vi "TOOLweb TRIGGER.vi"(4 "error in (no error)":errorcluster caption="Fehler (Eingang, kein Fehler)", 5 "IP-Adresse (localhost)":string="127.0.0.1", 7 "action":T2) -> (2 "trigger-Diagnose":T1, 3 "Trigger ausgeführt":bool)   [LabVIEW 2020, in "FT-IR.lvlib" / "TOOLweb Interface.lvlib"]
doc: "Ändert den Betriebszustand des Messgerätes durch Triggern einer Aktion \"action\" (start run, run once, stop run, pause run, resume run, take back). Der Trigger wird durch einen PollRequest an EVID 31..36 (je nach Aktion) ausgelöst. Nachher wird durch Polling der Variablen EVID30 (trigger-lastdatetime) verifiziert, ob der Trigger erfolgreich ausgeführt wurde.\n\n\"Trigger ausgeführt\" ist TRUE, wenn\n1) die Datum/Zeit in der Antwort einen Zeitpunkt nach dem Senden des PollRequests ergeben UND\n2) der Name der Aktion im Poll-Response mit der angeforderten Aktion übereinstimmt.\n\nDer Ausgangs-Cluster \"trigger-Diagnose\" ermöglicht eine weitere Fehlererkennung:\naction-name: die angeforderte Aktion\nlastname: die zuletzt erfolgreich ausgeführte Trigger-Aktion\nlastdatetime: der Zeitpunkt der zuletzt erfolgreich ausgeführten Aktion\nSystemzeit: der Zeitpunkt des Sendens der Trigger-Anforderung (PollRequest)"
uses:
  TOOLweb Interface.lvlib
  Trigger Aktionen.ctl
  Stoerungen/Stoerungen Messgeraet/Aktionen Kommunikation Stoerung.ctl
  TOOLweb Interface Hilfs-VIs.lvlib
  Stoerungen/Stoerungen.lvlib
  Typdefinitionen.lvlib
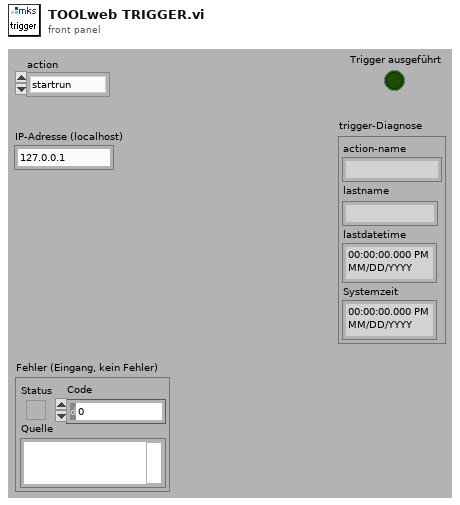
[diagram p1: front panel]
types:
  T1 = cluster{"action-name":string, "lastname":string, "lastdatetime":timestamp, "Systemzeit":timestamp}
  T2 = typedef "FT-IR.lvlib/TOOLweb Interface.lvlib/Typdefinitionen.lvlib/Trigger Aktionen.ctl" = enum16{"startrun", "runonce", "stoprun", "pauserun", "resumerun", "takeback"}
  T3 = typedef "Stoerungen.lvlib/Aktionen Kommunikation Stoerung.ctl" = enum16{"lesen", "init", "FT-IR Komm", "FT-IR Betriebsart", "FT-IR Hintergrund", "cRIO Komm", "PNS Komm", "Dichtheitstest", "Life Bit", "FTIR Komm AK", "PMA Komm", "FID Komm", "PMA Cal", "FID Ch4 Cal", "FID THC Cal", "Cal Timeout", "VFS 1 Komm", "VFS 2 Komm", "VFS 3 Komm", "VFS 4 Komm", "TRE 08 Komm", "CG-Test vorzeitig", "CG-Test Span 1", "CG-Test Span 2", "CG-Test Span 3", "CG-Test Messgas", "CG-Test löschen", "Test", "Amium AK", "AK Recept konfig", "AK Name konfig", "AK EKFG konfig"}
  T4 = enum16{"YYYYMMDD HH:MM:SS", "[YYMMDD][HH:MM:SS]"}
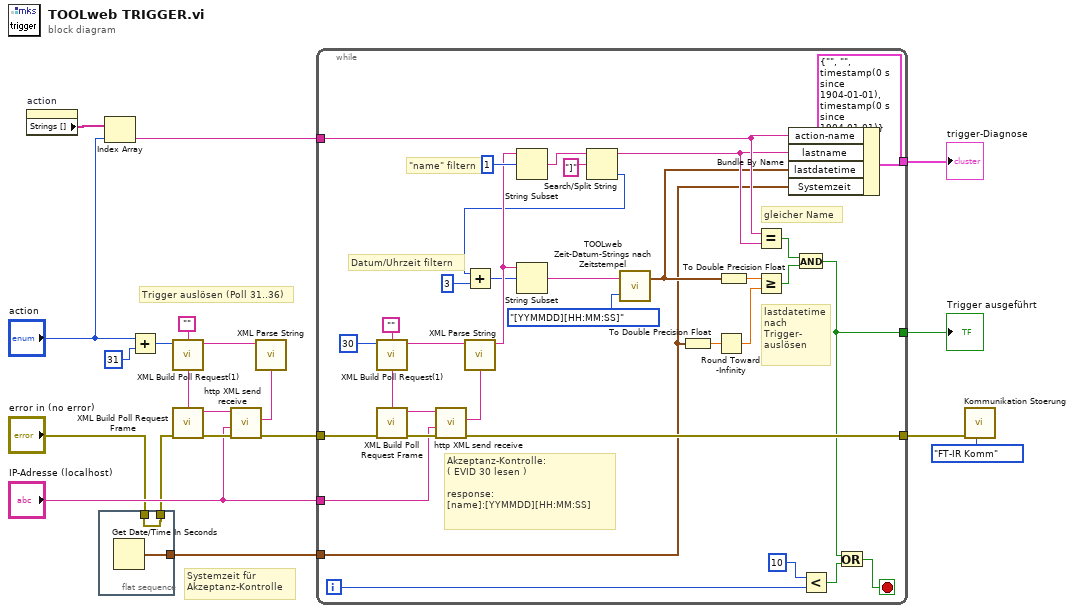
[diagram p0: block diagram]
diagram:
  # "Systemzeit für\nAkzeptanz-Kontrolle"
  # "Trigger auslösen (Poll 31..36)"
  n1 = property on="action" class="Enum (strikt)"() -> ("Strings []"=w14:string[])  [unwired: 2 in, 2 out]
  n2 = flat-sequence {
    tunnel: [w22] -> w5
    tunnel: "error in (no error)" -> [w21]
    tunnel: [w21] -> w3
    frame #0 {
      n3 = Get Date/Time In Seconds() -> (seconds since 1Jan1904=w22:timestamp)
    }
  }
  n4 = Index Array(array=w14, index="action") -> (element=w8:string)
  n5 = Add(x="action", y=31 ("EVID-Nummer")) -> (x+y=w12:i32)
  n6 = call "XML Build Poll Request(1).vi"("XML-Message alt"="", "EVID-Nummer"=w12) -> ("Attribut Name"=w16:string, "XML-Message neu"=w18:string)  [unwired: 6 out]
  n7 = call "XML Build Poll Request Frame.vi"("XML-Message"=w18, "error in (no error)"=w3) -> ("XML-Message fertig"=w19:string, "error out"=w20:errorcluster)  [unwired: 1 in, 5 out]
  n8 = call "http XML send receive.vi"("error in (no error)"=w20, "IP-Adresse (localhost)"="IP-Adresse (localhost)", "XML Request"=w19) -> ("error out"=w9:errorcluster, "Response Body (XML)"=w17:string)  [unwired: 3 out]
  n9 = call "XML Parse String.vi"("Attribut Name"=w16, "XML Response"=w17) -> ()  [unwired: 8 out]
  n10 = while {
    tunnel: [w52] -> w1
    tunnel: "IP-Adresse (localhost)" -> [w51]
    tunnel: w9 -> [w45]
    tunnel: w8 -> [w44]
    tunnel: [w40] -> w7
    tunnel: [w29] -> w6
    tunnel: w5 -> [w23]
    i -> [w39]
    stop <- w41 stop-if-true
    # "lastdatetime\nnach\nTrigger-\nauslösen"
    # "gleicher Name"
    # "Datum/Uhrzeit filtern"
    # "\"name\" filtern"
    # "Akzeptanz-Kontrolle:\n( EVID 30 lesen )\n\nresponse:\n[name]:[YYMMDD][HH:MM:SS]"
    n11 = call "XML Build Poll Request(1).vi"("XML-Message alt"="", "EVID-Nummer"=30) -> ("Attribut Name"=w53:string, "XML-Message neu"=w50:string)  [unwired: 6 out]
    n12 = call "XML Build Poll Request Frame.vi"("XML-Message"=w50, "error in (no error)"=w45) -> ("XML-Message fertig"=w57:string, "error out"=w56:errorcluster)  [unwired: 1 in, 5 out]
    n13 = call "http XML send receive.vi"("error in (no error)"=w56, "IP-Adresse (localhost)"=w51, "XML Request"=w57) -> ("error out"=w52:errorcluster, "Response Body (XML)"=w49:string)  [unwired: 3 out]
    n14 = call "XML Parse String.vi"("Attribut Name"=w53, "XML Response"=w49) -> ("Wert-String"=w36:string)  [unwired: 7 out]
    n15 = String Subset(string=w36, offset (0)=1 ("Offset (0)")) -> (substring=w47:string)  [unwired: 1 out]
    n16 = Search/Split String(string=w47, search string/char (-)="]" ("Nach String/Zeichen suchen (-)")) -> (substring before match=w43:string, offset of match=w34:i32)  [unwired: 2 out]
    n17 = Add(x=w34, y=3) -> (x+y=w35:i32)
    n18 = String Subset(string=w36, offset (0)=w35) -> (substring=w32:string)  [unwired: 1 out]
    n19 = call "TOOLweb Zeit-Datum-Strings nach Zeitstempel.vi"("Format"=T4."[YYMMDD][HH:MM:SS]", "Zeit/Datum-String"=w32) -> ("Zeitstempel"=w25:timestamp)  [unwired: 1 out]
    n20 = To Double Precision Float(number=w23) -> (double precision float=w27:dbl)
    n21 = Round Toward -Infinity(1:w27) -> (0:w26:dbl)
    n22 = To Double Precision Float(number=w25) -> (double precision float=w24:dbl)
    n23 = Equal?(x=w44, y=w43) -> (x = y?=w42:bool)
    n24 = Greater Or Equal?(x=w24, y=w26) -> (x >= y?=w28:bool)
    n25 = Bundle By Name(cluster=T1 {"action-name"="", "lastname"="", "lastdatetime"=timestamp(0 s since 1904-01-01), "Systemzeit"=timestamp(0 s since 1904-01-01)} ("trigger-Diagnose"), "action-name"=w44, "lastname"=w43, "lastdatetime"=w25, "Systemzeit"=w23) -> (w29:T1)
    n26 = And(x=w42, y=w28) -> (x .and. y?=w40:bool)
    n27 = Less?(x=10, y=w39) -> (x < y?=w38:bool)
    n28 = Or(x=w40, y=w38) -> (x .or. y?=w41:bool)
  }
  "trigger-Diagnose" <- w6
  "Trigger ausgeführt" <- w7
  n29 = call "Kommunikation Stoerung.vi"("Aktionen"=Aktionen_Kommunikation_Stoerung."FT-IR Komm", "error in"=w1) -> ()  [unwired: 9 in, 1 out]
